vi "T-periodic Power Exponential Function.vi"(6 "L":i32 caption="Order L", 8 "Error In":errorcluster, 9 "T":dbl caption="Period T", 10 "tau":dbl caption="Lifetime tau", 11 "x":dbl caption="Variable x") -> (0 "Error Out":errorcluster, 3 "f_L,tau,T(x)":dbl)   [LabVIEW 2021, in "Math.lvlib"]
uses:
  449d7667-511f-401a-ba57-ebd09ba8ed3f.vi
  Math.lvlib
  <vilib>/gmath/NI_Gmath.lvlib
  Error/Error.lvlib
  Time/Time.lvlib
panel:
  out "Time (s)":dbl
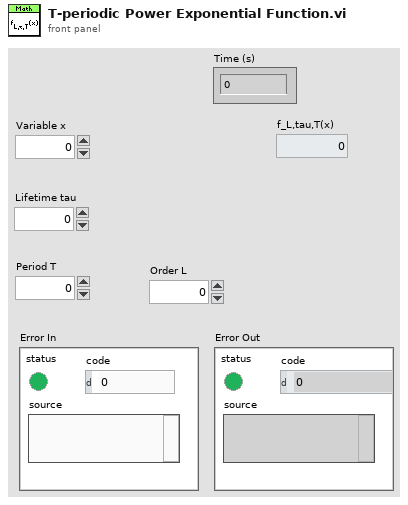
[diagram p1: front panel]
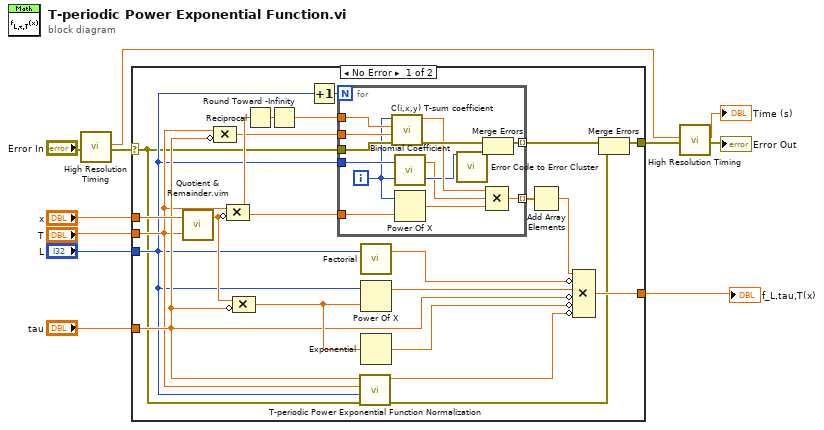
[diagram p0: block diagram]
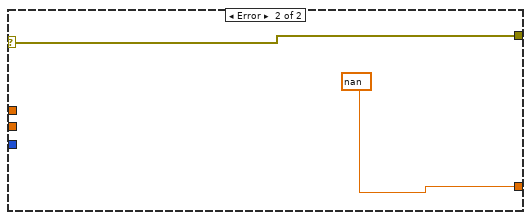
[diagram p2: hidden frame]
diagram:
  n1 = call "High Resolution Timing.vi"("Error In"="Error In") -> ("elapsed (relative) seconds"=w2:dbl, "Error Out"=w4:errorcluster)  [unwired: 16 in, 1 out]
  n2 = case shown="No Error" w4 {
    selector: w4 -> [w14 w49]
    tunnel: "tau" -> [w17 _]
    tunnel: "L" -> [w15 _]
    tunnel: "T" -> [w16 _]
    tunnel: "x" -> [w28 _]
    tunnel: [w26 w49] -> w6
    tunnel: [w21 nan] -> w5
    frame No Error {
      n3 = call "Quotient & Remainder.vim"("y"=w16, "x"=w28) -> ("x - E(x/y)y"=w20:dbl)  [unwired: 1 out]
      n4 = Compound Arithmetic op=MULTIPLY(w16, invert w17) -> (w18:dbl)
      n5 = Compound Arithmetic op=MULTIPLY(w16, invert w20) -> (w25:dbl)
      n6 = Compound Arithmetic op=MULTIPLY(w20, invert w17) -> (w31:dbl)
      n7 = Reciprocal(x=w25) -> (1/x=w24:dbl)
      n8 = Round Toward -Infinity(1:w24) -> (0:w23:dbl)
      n9 = Increment(x=w15) -> (x+1=w29:i32)
      n10 = for {
        N: w29 -> [_]
        tunnel: w15 -> [w35]
        tunnel: w25 -> [w47]
        tunnel: [w41] -> w27 mode=indexing
        tunnel: w14 -> [w36]
        tunnel: w23 -> [w45]
        tunnel: w18 -> [w44]
        tunnel: [w39] -> w22 mode=indexing
        i -> [w34]
        n11 = call "C(i,x,y) T-sum coefficient.vi"("Error In"=w36, "y"=w44, "x"=w45, "i"=w34) -> ("Error Out"=w46:errorcluster, "C(i, x, y)"=w43:dbl)  [unwired: 6 in]
        n12 = call <vilib>:"Binomial Coefficient.vi"("k"=w34, "n"=w35) -> ("error"=w42:i32, "binomial coefficient (n,k)"=w37:dbl)
        n13 = Power Of X(1:w47, 2:w34) -> (0:w38:dbl)
        n14 = call "Error Code to Error Cluster.vi"("Error Code"=w42) -> ("Error Out"=w40:errorcluster)  [unwired: 14 in]
        n15 = Merge Errors(w46, w40) -> (w41:errorcluster)
        n16 = Compound Arithmetic op=MULTIPLY(w43, w37, w38) -> (w39:dbl)
      }
      n17 = call "T-periodic Power Exponential Function Normalization.vi"("Error In"=w14, "L"=w15, "T"=w16, "tau"=w17) -> ("Error Out"=w12:errorcluster, "N(L,tau,T)"=w13:dbl)  [unwired: 6 in]
      n18 = call <vilib>:"Factorial.vi"("n"=w15) -> ("n!"=w33:dbl)  [unwired: 2 in]
      n19 = Power Of X(1:w31, 2:w15) -> (0:w32:dbl)
      n20 = Exponential(1:w31) -> (0:w30:dbl)
      n21 = Add Array Elements(numeric array=w22) -> (sum=w19:dbl)
      n22 = Compound Arithmetic op=MULTIPLY(w19, invert w33, w32, invert w17, invert w30, invert w13) -> (w21:dbl)
      n23 = Merge Errors(w27, w12) -> (w26:errorcluster)
    }
    frame Error {
    }
  }
  "f_L,tau,T(x)" <- w5
  n24 = call "High Resolution Timing.vi"("relative seconds (NaN)"=w2, "Error In"=w6) -> ("elapsed (relative) seconds"=→"Time (s)":dbl, "Error Out"=→"Error Out":errorcluster)  [unwired: 15 in, 1 out]
